vi "TESTE CURVA GRUPO-3.vi"() -> ()   [LabVIEW 2014]
uses:
  <vilib>/Platform/TimedLoop/XDataNode/timing_clust.ctl
  <vilib>/Platform/TimedLoop/XDataNode/nitl_modes.ctl
  <vilib>/Platform/TimedLoop/XDataNode/wakeup.ctl
  <vilib>/Platform/TimedLoop/XDataNode/XDataNode.xnode
  <userlib>/Newport ESP301/Newport ESP301.lvlib
  <vilib>/Platform/TimedLoop/XDataNode/XDNodeRunTimeDep.lvlib
panel:
  in  "arc sweep angle":dbl=360.0 format="%#_13g"
  in  "Second coordonate of arc center":dbl format="%#_13g"
  in  "first coordonate of arc":dbl=0.1 format="%#_13g"
  in  "Stop Button":bool
  out "error out":errorcluster
  out "X (mm)":dbl=0.001 format="%.2g"
  out "Y (um)":dbl=0.0005 format="%.1f"
  out "XY Graph":cluster{dbl[], dbl[]}(graph)
  in  "Refresh Button":bool
  in  "Velocity":dbl=0.1
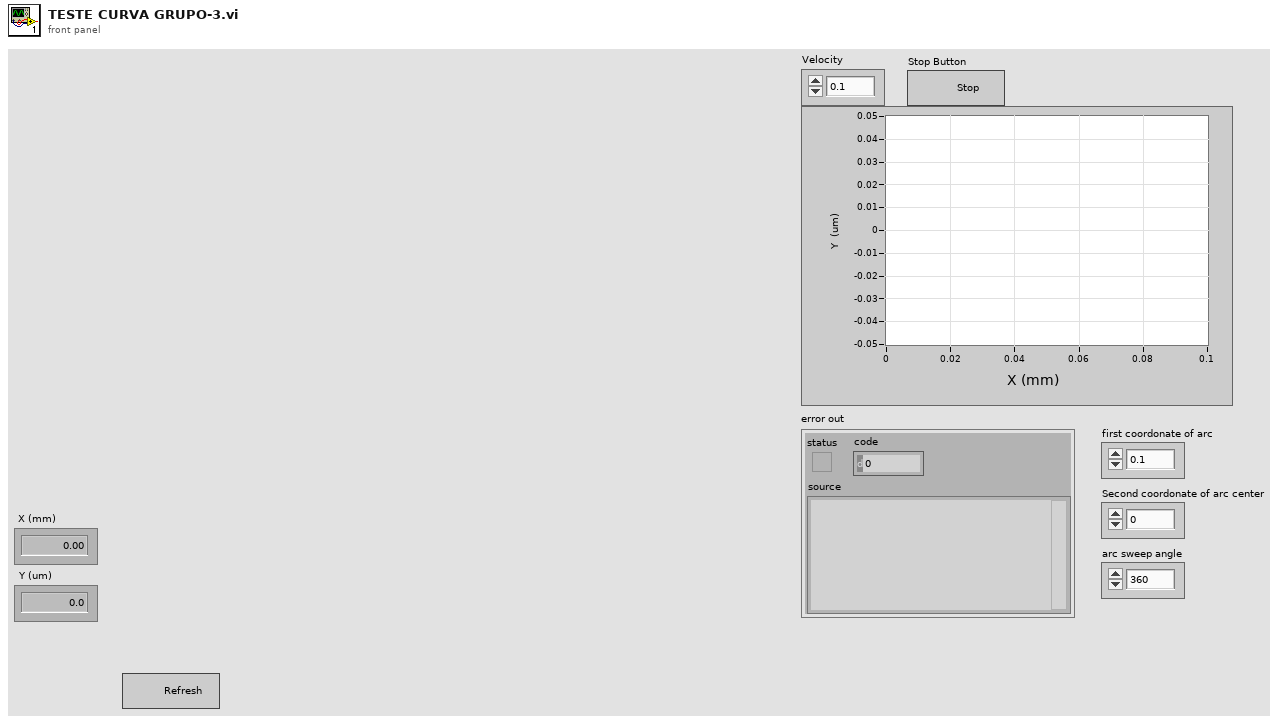
[diagram p1: front panel]
types:
  T1 = typedef "XDNodeRunTimeDep.lvlib/timing_clust.ctl" = cluster{"Expected End [f-1]":u64, "Actual End [f-1]":u64, "Finished Late? [f-1]":bool, "Expected End [i-1]":u64, "Actual End [i-1]":u64, "Finished Late? [i-1]":bool, "Expected Start [i]":u64, "Actual Start [i]":u64, "Expected Start [f]":u64, "Actual Start [f]":u64, "Source Name":string, "Structure Name":string, "Period":i64, "Deadline":i64, "Offset":i64, "Start":i64, "Priority":i32, "Timeout":i32, "Mode":T2, "Wakeup Reason":T3, "Error":errorcluster, "Source Type":string, "Secondary Source Type":string, "Global End Time":u64, "Global Start Time":u64, "Frame Duration":u64, "Iteration Duration":u64, "Assigned CPU":i32, "I/O Scan Engine Mode":u32}
  T2 = typedef "XDNodeRunTimeDep.lvlib/nitl_modes.ctl" = enum32{"No Change", "Process missed periods, maintain original phase", "Discard missed periods, maintain original phase", "Process missed periods, ignore original phase", "Discard missed periods, ignore original phase"}
  T3 = typedef "XDNodeRunTimeDep.lvlib/wakeup.ctl" = enum32{"Normal", "Aborted", "Asynchronous wakeup", "Timing source error", "Timed loop error", "Timeout"}
  T4 = cluster{"first coordonate of arc":dbl, "Second coordonate of arc center":dbl, "arc sweep angle":dbl}
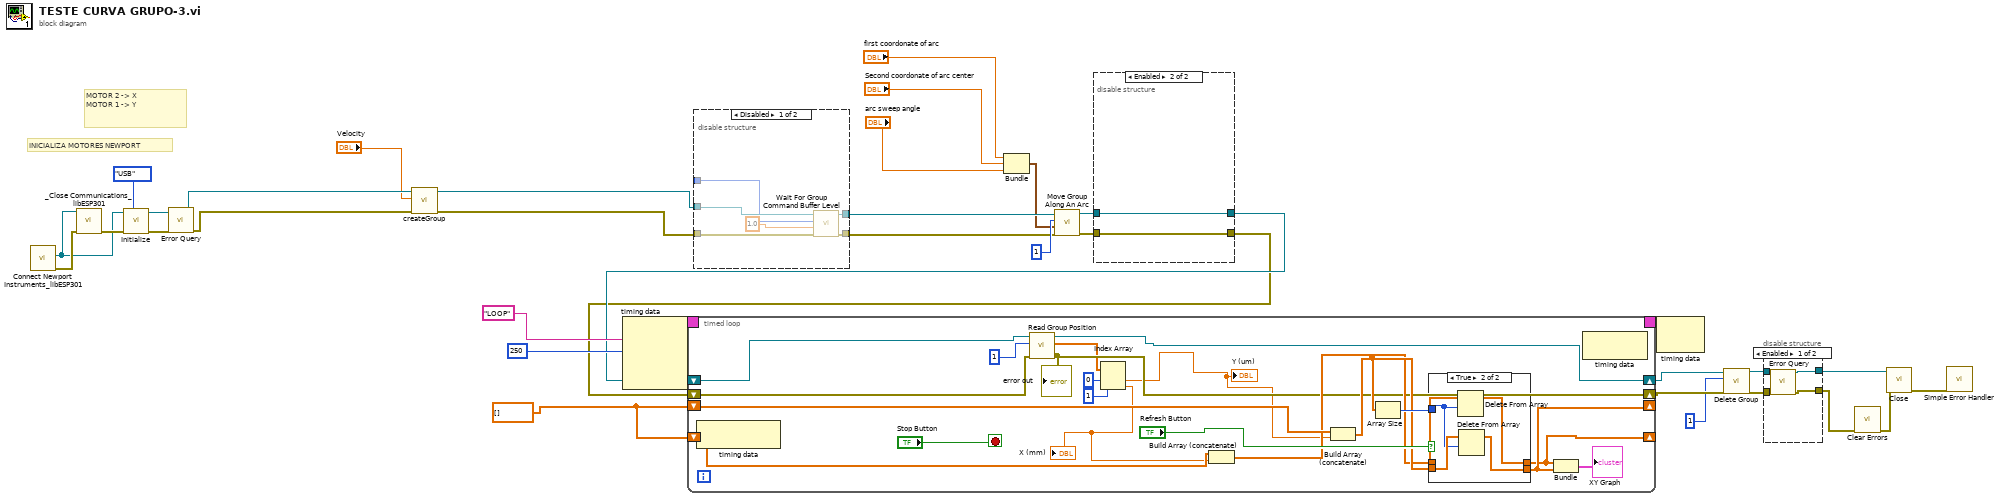
[diagram p0: block diagram]
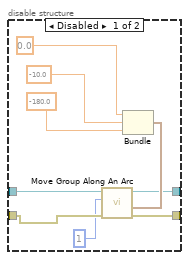
[diagram p2: hidden frame]
diagram:
  w13 = dbl[] []
  # "MOTOR 2 -> X\nMOTOR 1 -> Y"
  # "INICIALIZA MOTORES NEWPORT"
  n1 = call <userlib>:"Connect Newport Instruments_libESP301.vi"() -> ("error (duplicate)"=w34:errorcluster, "VISA resource name (duplicate)"=w33:refnum<visa-resource-name>)  [unwired: 7 in, 3 out]
  n2 = call <userlib>:"_Close Communications_libESP301.vi"("Instrument Channel"=w33, "error in (no error)"=w34) -> ("error out"=w36:errorcluster)  [unwired: 13 in]
  n3 = call <userlib>:"Initialize.vi"("VISA resource name"=w33, "error in (no error)"=w36, "Serial Link (RS232)"=enum16{"RS232", "USB"}."USB") -> ("VISA resource name out"=w32:refnum<visa-resource-name>, "error out"=w31:errorcluster)  [unwired: 6 in]
  n4 = call <userlib>:"Error Query.vi"("error in (no error)"=w31, "VISA resource name"=w32) -> ("error out"=w29:errorcluster, "VISA resource name out"=w30:refnum<visa-resource-name>)  [unwired: 2 in, 2 out]
  n5 = call "createGroup.vi"("error in (no error)"=w29, "Velocity"="Velocity", "VISA Refnum in"=w30) -> ("error out"=w26:errorcluster, "VISA Refnum out"=w27:refnum<visa-resource-name>)  [unwired: 7 in]
  n6 = node-c288("LOOP" ("Structure Name"), i64 250 ("Period")) -> (w17:T1)  [unwired: 2 in]
  n7 = disable-structure shown="Disabled" {
    disable-tunnel: w27 -> [w42 w44]
    disable-tunnel: w26 -> [w41 w43]
    disable-tunnel: [w40 w44] -> w25
    disable-tunnel: [w39 w43] -> w24
    disable-tunnel: _ -> [w37 _]
    frame Disabled {
      n8 = call <userlib>:"Wait For Group Command Buffer Level.vi"("error in (no error)"=w41, "level in group via point buffer"=1.0, "Group Number (1)"=w37, "VISA resource name"=w42) -> ("error out"=w39:errorcluster, "VISA resource name out"=w40:refnum<visa-resource-name>)  [unwired: 2 in]
    }
    frame Enabled {
    }
  }
  n9 = Bundle("first coordonate of arc"="first coordonate of arc", "Second coordonate of arc center"="Second coordonate of arc center", "arc sweep angle"="arc sweep angle") -> (w18:T4)  [unwired: 1 in]
  n10 = call <userlib>:"Move Group Along An Arc.vi"("error in (no error)"=w24, "Arc  Parameters"=w18, "Group Number (1)"=1, "VISA resource name"=w25) -> ("error out"=w22:errorcluster, "VISA resource name out"=w23:refnum<visa-resource-name>)  [unwired: 2 in]
  n11 = disable-structure shown="Enabled" {
    disable-tunnel: w23 -> [w53 w55]
    disable-tunnel: w22 -> [w52 w54]
    disable-tunnel: [w46 w55] -> w8
    disable-tunnel: [w45 w54] -> w7
    frame Disabled {
      n12 = Bundle(0.0, -10.0, -180.0) -> (w48:cluster{dbl, dbl, dbl})  [unwired: 1 in]
      n13 = call <userlib>:"Move Group Along An Arc.vi"("error in (no error)"=w52, "Arc  Parameters"=w48, "Group Number (1)"=1, "VISA resource name"=w53) -> ("error out"=w45:errorcluster, "VISA resource name out"=w46:refnum<visa-resource-name>)  [unwired: 2 in]
    }
    frame Enabled {
    }
  }
  n14 = timed-loop {
    timing: w17 -> [_]
    timing-out: [_] -> w16
    shift-right: [w63] -> w6
    shift-left: w8 -> [w65]
    shift-right: [w62] -> w5
    shift-left: w7 -> [w64]
    shift-right: [w68] -> _
    shift-left: w13 -> [w72]
    shift-right: [w67] -> _
    shift-left: w13 -> [w70]
    stop <- "Stop Button" stop-if-true
    n15 = node-c288() -> ()  [unwired: 1 in, 1 out]
    n16 = call <userlib>:"Read Group Position.vi"("error in (no error)"=w64, "Group Number (1)"=1, "VISA resource name"=w65) -> ("error out"=w62:errorcluster, "Position (units)"=w59:dbl[], "VISA resource name out"=w63:refnum<visa-resource-name>)  [unwired: 2 in]
    "error out" <- w62
    n17 = Index Array(array=w59, index #1=0 ("index"), index #2=1 ("index")) -> (element #1=w58:dbl, element #2=w57:dbl)
    "X (mm)" <- w57
    "Y (um)" <- w58
    n18 = Build Array (concatenate)(w70, w57) -> (w69:dbl[])
    n19 = Build Array (concatenate)(w72, w58) -> (w71:dbl[])
    n20 = Array Size(array=w71) -> (size(s)=w73:i32)
    n21 = case shown="True" "Refresh Button" {
      tunnel: [w77 w79] -> w67
      tunnel: w69 -> [w77 w82]
      tunnel: [w76 w78] -> w68
      tunnel: w71 -> [w76 w81]
      tunnel: w73 -> [_ w80]
      frame False {
      }
      frame True {
        n22 = Delete From Array(array=w82, length=w80) -> (array with subset deleted=w79:dbl[])  [unwired: 1 in, 1 out]
        n23 = Delete From Array(array=w81, length=w80) -> (array with subset deleted=w78:dbl[])  [unwired: 1 in, 1 out]
      }
    }
    n24 = Bundle(w67, w68) -> (→"XY Graph":cluster{dbl[], dbl[]})  [unwired: 1 in]
    n25 = node-c288() -> ()  [unwired: 1 in, 1 out]
  }
  n26 = node-c288(w16) -> ()  [unwired: 1 out]
  n27 = call <userlib>:"Delete Group.vi"("error in (no error)"=w5, "Group Number (1)"=1, "VISA resource name"=w6) -> ("error out"=w11:errorcluster, "VISA resource name out"=w12:refnum<visa-resource-name>)  [unwired: 3 in]
  n28 = disable-structure shown="Enabled" {
    disable-tunnel: w12 -> [w88 w90]
    disable-tunnel: w11 -> [w87 w89]
    disable-tunnel: [w86 w90] -> w10
    disable-tunnel: [w85 w89] -> w3
    frame Enabled {
      n29 = call <userlib>:"Error Query.vi"("error in (no error)"=w87, "VISA resource name"=w88) -> ("error out"=w85:errorcluster, "VISA resource name out"=w86:refnum<visa-resource-name>)  [unwired: 2 in, 2 out]
    }
    frame Disabled {
    }
  }
  n30 = call <vilib>:"Clear Errors.vi"("error in (no error)"=w3) -> ("error out"=w2:errorcluster)  [unwired: 5 in, 1 out]
  n31 = call <userlib>:"Close.vi"("error in (no error)"=w2, "VISA resource name"=w10) -> ("error out"=w9:errorcluster)  [unwired: 9 in]
  n32 = call <vilib>:"Simple Error Handler.vi"("error in (no error)"=w9) -> ()  [unwired: 4 in, 5 out]
